vi "dataconvert_array.vi"(7 "输入的TTL信号序列":i32[](array[numeric])=[5, 0, -1, 1, 0, 0, 0, 0, 0], 8 "总时间（ms）":i32=10, 9 "相乘倍数":i32=1) -> (2 "输出编码后的TTL序列":i32[](array[numeric]))   [LabVIEW 2021]
panel:
  in  "Numeric":i32
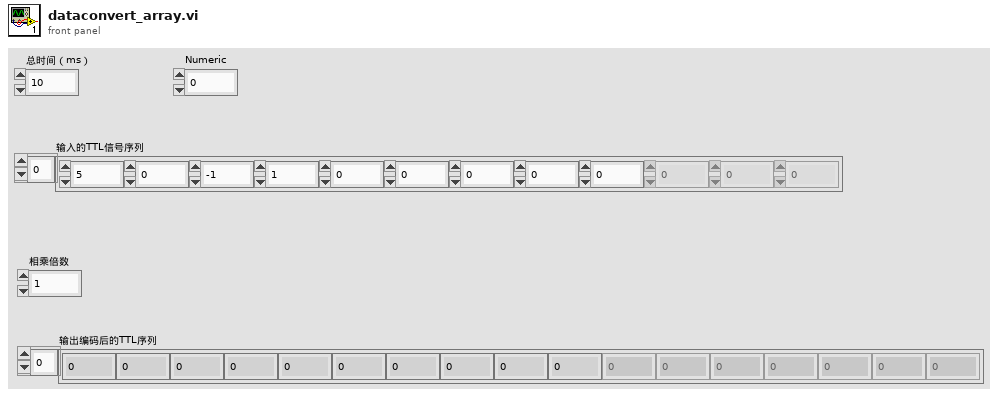
[diagram p1: front panel]
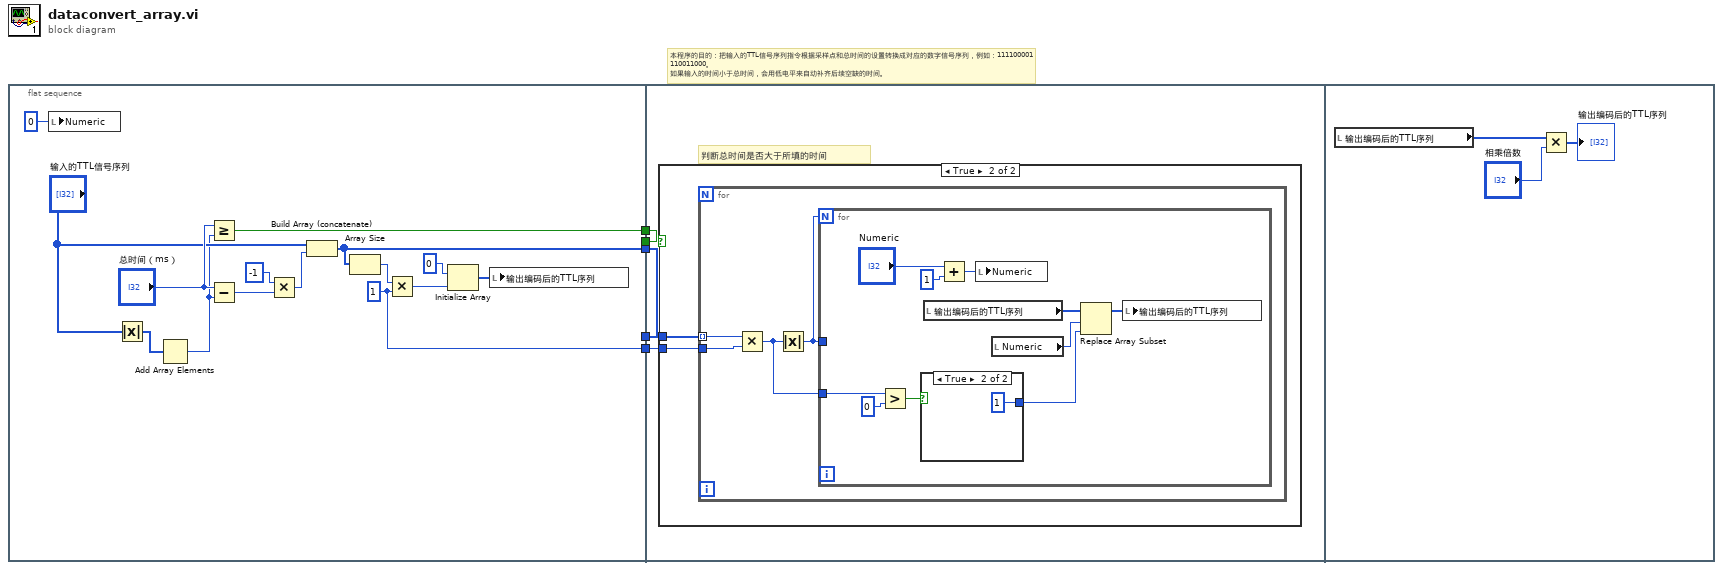
[diagram p0: block diagram]
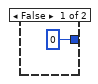
[diagram p3: hidden frame]
diagram:
  # "本程序的目的：把输入的TTL信号序列指令根据采样点和总时间的设置转换成对应的数字信号序列，例如：111100001110011000。\n如果输入的时间小于总时间，会用低电平来自动补齐后续空缺的时间。"
  n1 = flat-sequence {
    tunnel: [w9] -> w3
    tunnel: [w8] -> w2
    tunnel: [w7] -> w1
    tunnel: w3 -> [w21]
    tunnel: w2 -> [w20]
    tunnel: w1 -> [w19]
    frame #0 {
      w8 = 1 ("每毫秒采样点")
      n2 = local write "Numeric"(0 ("Numeric")) -> ()
      n3 = Absolute Value(x="输入的TTL信号序列") -> (abs(x)=w5:i32[])
      n4 = Add Array Elements(numeric array=w5) -> (sum=w4:i32)
      n5 = Greater Or Equal?(x="总时间（ms）", y=w4) -> (x >= y?=w7:bool)
      n6 = Subtract(x="总时间（ms）", y=w4) -> (x-y=w13:i32)
      n7 = Multiply(x=-1, y=w13) -> (x*y=w14:i32)
      n8 = Build Array (concatenate)("输入的TTL信号序列", w14) -> (w9:i32[])
      n9 = Array Size(array=w9) -> (size(s)=w15:i32)
      n10 = Multiply(x=w15, y=w8) -> (x*y=w16:i32)
      n11 = Initialize Array(0 ("element"), w16) -> (w17:i32[])
      n12 = local write "输出编码后的TTL序列"(w17) -> ()
    }
    frame #1 {
      # "判断总时间是否大于所填的时间"
      n13 = case shown="True" w19 {
        tunnel: w21 -> [_ w23]
        tunnel: w20 -> [_ w22]
        frame False {
        }
        frame True {
          n14 = for {
            tunnel: w23 -> [w26] mode=indexing
            tunnel: w22 -> [w27]
            n15 = Multiply(x=w26, y=w27) -> (x*y=w25:i32)
            n16 = Absolute Value(x=w25) -> (abs(x)=w24:i32)
            n17 = for {
              N: w24 -> [_]
              tunnel: w25 -> [w35]
              tunnel: w24 -> [_]
              n18 = Greater?(x=w35, y=i16 0) -> (0:w37:bool)
              n19 = case shown="True" w37 {
                tunnel: [i16 0 i16 1] -> w32
                frame False {
                }
                frame True {
                }
              }
              n20 = local read "输出编码后的TTL序列"() -> (w33:i32[])
              n21 = Add(x="Numeric", y=1) -> (x+y=w29:i32)
              n22 = local write "Numeric"(w29) -> ()
              n23 = local read "Numeric"() -> (w28:i32)
              n24 = Replace Array Subset(array=w33, new element=w32, index=w28) -> (w34:i32[])
              n25 = local write "输出编码后的TTL序列"(w34) -> ()
            }
          }
        }
      }
    }
    frame #2 {
      n26 = local read "输出编码后的TTL序列"() -> (w42:i32[])
      n27 = Multiply(x=w42, y="相乘倍数") -> (x*y=→"输出编码后的TTL序列":i32[])
    }
  }
